vi "Read Conversion Time.vi"(8 "error in":errorcluster, 11 "AI with conversion filter channel in":refnum<class "AI with Conversion Filter Channel.lvclass">) -> (0 "error out":errorcluster, 2 "conversion time":T1, 3 "AI with conversion filter channel out":refnum<class "AI with Conversion Filter Channel.lvclass">)   [LabVIEW 2017, in "Scan Engine Scripting.lvlib" / "AI with Conversion Filter Channel.lvclass"]
uses:
  AI with Conversion Filter Channel.lvclass
  Conversion Time.ctl
  AI with Conversion Filter Channel.lvclass/AI with Conversion Filter Channel.ctl
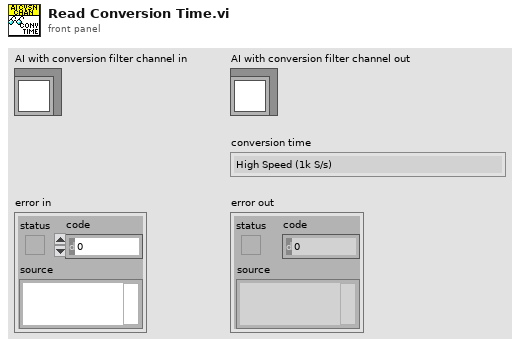
[diagram p1: front panel]
types:
  T1 = typedef "Scan Engine Scripting.lvlib/AI with Conversion Filter Channel.lvclass/Conversion Time.ctl" = enum16{"High Speed (1k S/s)", "Medium Speed (100 S/s)", "Medium Resolution (50/60 Hz Rejection - 12 S/s)", "High Resolution (50/60 Hz Rejection - 2 S/s)"}
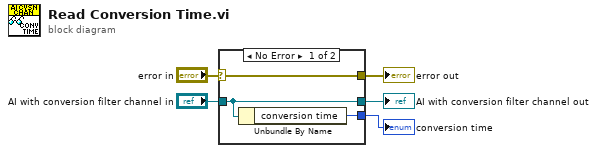
[diagram p0: block diagram]
diagram:
  n1 = case shown="No Error" "error in" {
    selector: "error in" -> [w8 w9]
    tunnel: [w8 w9] -> w4
    tunnel: [w7 w10] -> w2
    tunnel: "AI with conversion filter channel in" -> [w7 w10]
    tunnel: [w6 _] -> w1
    frame No Error {
      n2 = Unbundle By Name(w7) -> ("conversion time"=w6:T1)
    }
    frame Error {
    }
  }
  "error out" <- w4
  "AI with conversion filter channel out" <- w2
  "conversion time" <- w1
